vi "chart series set categories lv.vi"(5 "last_col":u16, 6 "last_row":u32, 7 "first_col":u16, 8 "error in (no error)":errorcluster, 9 "first_row":u32, 10 "sheetname":string, 11 "series":u32) -> (0 "error out":errorcluster)   [LabVIEW 2015, in "xlsxwriter.lvlib"]
doc: "void chart_series_set_categories_lv(lxw_chart_series series, const char *sheetname, lxw_row_t first_row, lxw_col_t first_col, lxw_row_t last_row, lxw_col_t last_col);"
uses:
  xlsxwriter.lvlib
  xlsxwriter.dll
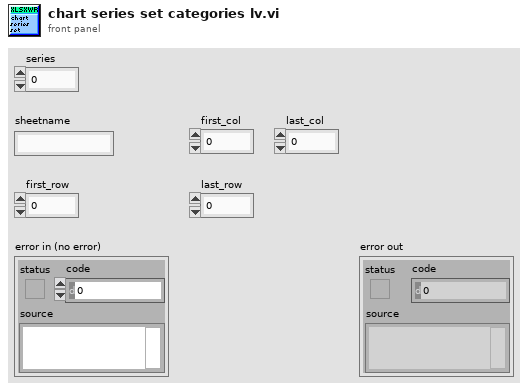
[diagram p1: front panel]
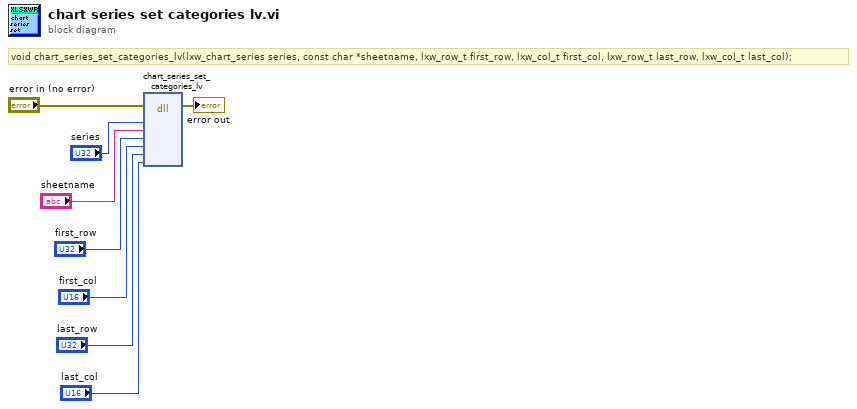
[diagram p0: block diagram]
diagram:
  # "void chart_series_set_categories_lv(lxw_chart_series series, const char *sheetname, lxw_row_t first_row, lxw_col_t first_col, lxw_row_t last_row, lxw_col_t last_col);"
  n1 = dll-call lib="C:/Users/WDAGUtilityAccount/Desktop/lv_vis_added_cell/xlsxwriter.*" fn="chart_series_set_categories_lv"(error in="error in (no error)", "series"="series", "sheetname"="sheetname", "first_row"="first_row", "first_col"="first_col", "last_row"="last_row", "last_col"="last_col") -> (error out=→"error out":errorcluster)  [unwired: 9 in, 1 out]
